vi "Adjust_Seconds_xRef.vi"(9 "Coords":T1, 11 "CtlRef":refnum<vi>) -> ()   [LabVIEW 2016]
uses:
  <vilib>/Utility/miscctls.llb/LVPoint32TypeDef.ctl
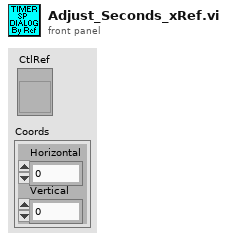
[diagram p1: front panel]
types:
  T1 = typedef "LVPoint32TypeDef.ctl" = cluster{"Horizontal":i32, "Vertical":i32}
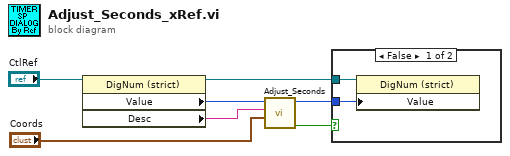
[diagram p0: block diagram]
diagram:
  n1 = property class="DigNum (strict)"(reference="CtlRef") -> (reference out=w6:refnum<vi>, "Value"=w5:i32, "Desc"=w3:string)  [unwired: 1 in, 1 out]
  n2 = call "Adjust_Seconds.vi"("Coords"="Coords", "Label"=w3, "Seconds"=w5) -> ("Cancelled"=w7:bool, "Seconds_out"=w4:i32)  [unwired: 7 in]
  n3 = case shown="False" w7 {
    tunnel: w4 -> [w8 _]
    tunnel: w6 -> [w9 _]
    frame False {
      n4 = property class="DigNum (strict)"(reference=w9, "Value"=w8) -> ()  [unwired: 1 in, 2 out]
    }
    frame True {
    }
  }
